vi "Read intensity.vi"(8 "error in (no error)":errorcluster, 11 "State in":refnum<class "State.lvclass">) -> (0 "error out":errorcluster, 2 "intensity":dbl[](array[numeric]), 3 "State out":refnum<class "State.lvclass">)   [LabVIEW 2016, in "State.lvclass"]
uses:
  State.lvclass
  State.lvclass/State.ctl
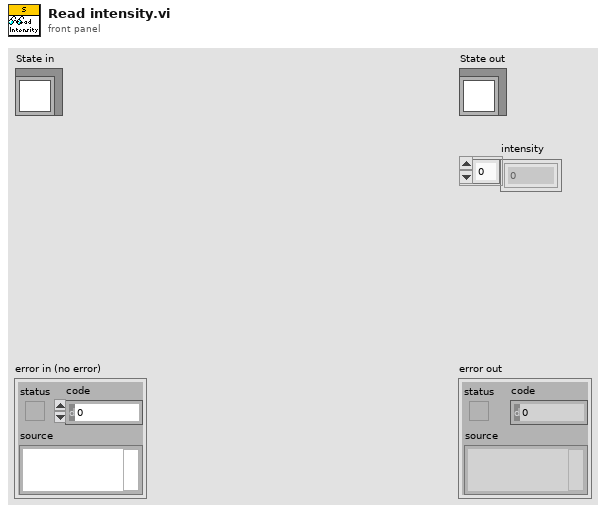
[diagram p1: front panel]
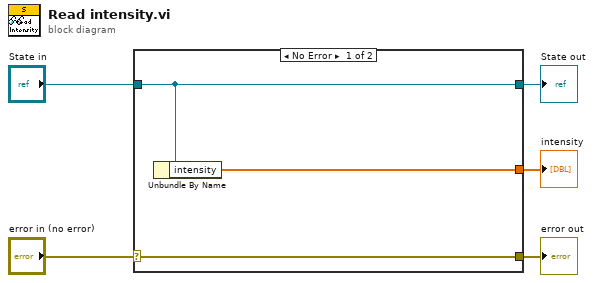
[diagram p0: block diagram]
diagram:
  n1 = case shown="No Error" "error in (no error)" {
    selector: "error in (no error)" -> [w8 w9]
    tunnel: [w8 w9] -> w4
    tunnel: [w7 w10] -> w2
    tunnel: "State in" -> [w7 w10]
    tunnel: [w6 _] -> w1
    frame No Error {
      n2 = Unbundle By Name(w7) -> ("intensity"=w6:dbl[])
    }
    frame Error {
    }
  }
  "error out" <- w4
  "State out" <- w2
  "intensity" <- w1
